vi "I2C Write.vi"(9 "data":u8, 10 "intAddress":u8, 11 "deviceID":u8) -> (3 "function return":u32)   [LabVIEW 2018, in "AndorSDK.lvlib"]
doc: "EXPNETTYPE unsigned int WINAPI I2CWrite(BYTE deviceID, BYTE intAddress, BYTE data);"
uses:
  AndorSDK.lvlib
  ATMCD32D.dll
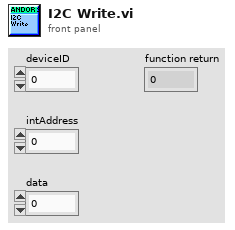
[diagram p1: front panel]
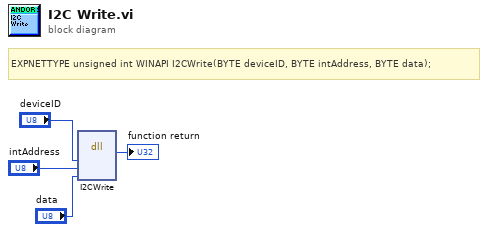
[diagram p0: block diagram]
diagram:
  # "EXPNETTYPE unsigned int WINAPI I2CWrite(BYTE deviceID, BYTE intAddress, BYTE data);"
  n1 = dll-call lib="PTH2babs E\nPersönliches02 - Arbeit03-HiwijobsLabviewCodelibANDOR\tAndor SDK\nATMCD32D.*" fn="I2CWrite"("deviceID"="deviceID", "intAddress"="intAddress", "data"="data") -> (→"function return":u32)  [unwired: 6 in, 2 out]
